vi "Initial_guess_gaussian_fit.vi"(10 "x-Axis in":dbl[](array[numeric]), 11 "Signal in":dbl[](array[numeric])) -> (0 "Initial guess FWHM":dbl, 1 "Initial guess Sigma":dbl, 2 "x-Axis out":dbl[](array[numeric]), 3 "Signal out":dbl[](array[numeric]), 4 "Parameter Bounds Cluster":T1, 5 "Initial Guess Cluster":T2, 6 "Initial guess Amplitude":dbl, 8 "Initial guess Offset":dbl)   [LabVIEW 2018]
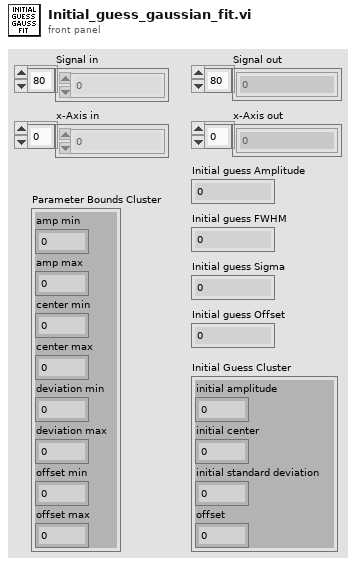
[diagram p1: front panel]
types:
  T1 = cluster{"amp min":dbl, "amp max":dbl, "center min":dbl, "center max":dbl, "deviation min":dbl, "deviation max":dbl, "offset min":dbl, "offset max":dbl}
  T2 = cluster{"initial amplitude":dbl, "initial center":dbl, "initial standard deviation":dbl, "offset":dbl}
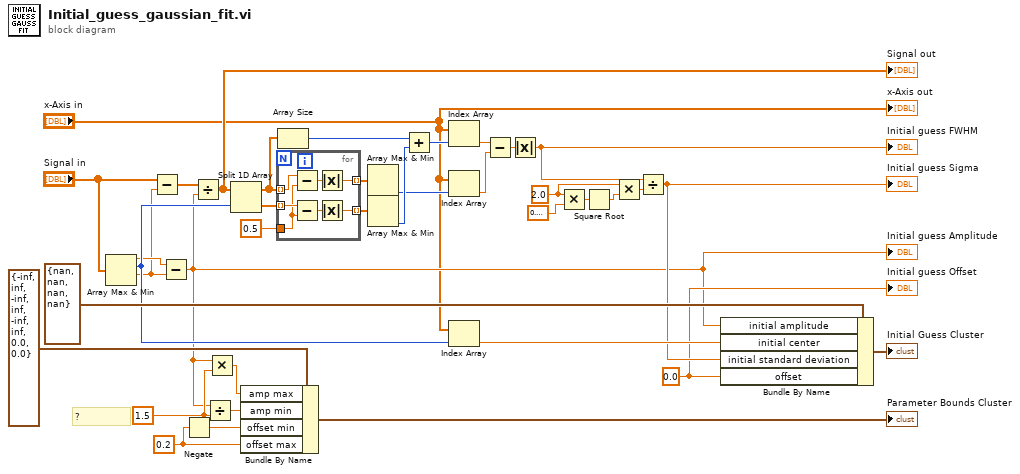
[diagram p0: block diagram]
diagram:
  w5 = 0.2 ("offset min")
  w8 = 1.5
  w11 = 0.0
  w36 = 2.0 ("x")
  # "?"
  n1 = Array Max & Min(array="Signal in") -> (max value=w14:dbl, max index (indices)=w20:i32, min value=w13:dbl)  [unwired: 1 out]
  n2 = Subtract(x="Signal in", y=w13) -> (x-y=w12:dbl[])
  n3 = Subtract(x=w14, y=w13) -> (x-y=w3:dbl)
  "Initial guess Amplitude" <- w3
  n4 = Negate(x=w5) -> (-x=w4:dbl)
  n5 = Divide(x=w12, y=w3) -> (x/y=w10:dbl[])
  "Signal out" <- w10
  n6 = Divide(x=w3, y=w8) -> (x/y=w7:dbl)
  n7 = Multiply(x=w3, y=w8) -> (x*y=w6:dbl)
  n8 = Split 1D Array(array=w10, index=w20) -> (first subarray=w24:dbl[], second subarray=w25:dbl[])
  n9 = Bundle By Name(cluster=T1 {"amp min"=-inf, "amp max"=inf, "center min"=-inf, "center max"=inf, "deviation min"=-inf, "deviation max"=inf, "offset min"=0.0, "offset max"=0.0} ("parameter bounds"), "amp max"=w6, "amp min"=w7, "offset min"=w4, "offset max"=w5) -> (→"Parameter Bounds Cluster":T1)
  n10 = for {
    tunnel: [w44] -> w33 mode=indexing
    tunnel: w24 -> [w42] mode=indexing
    tunnel: w25 -> [w41] mode=indexing
    tunnel: [w40] -> w32 mode=indexing
    tunnel: 0.5 -> [w39]
    n11 = Subtract(x=w42, y=w39) -> (x-y=w43:dbl)
    n12 = Subtract(x=w41, y=w39) -> (x-y=w45:dbl)
    n13 = Absolute Value(x=w43) -> (abs(x)=w40:dbl)
    n14 = Absolute Value(x=w45) -> (abs(x)=w44:dbl)
  }
  n15 = Array Size(array=w24) -> (size(s)=w29:i32)
  n16 = Array Max & Min(array=w32) -> (min index (indices)=w26:i32)  [unwired: 3 out]
  n17 = Array Max & Min(array=w33) -> (min index (indices)=w28:i32)  [unwired: 3 out]
  n18 = Add(x=w29, y=w28) -> (x+y=w27:i32)
  n19 = Index Array(array="x-Axis in", index=w27) -> (element=w22:dbl)
  n20 = Index Array(array="x-Axis in", index=w26) -> (element=w23:dbl)
  n21 = Index Array(array="x-Axis in", index=w20) -> (element=w19:dbl)
  n22 = Subtract(x=w22, y=w23) -> (x-y=w31:dbl)
  n23 = Absolute Value(x=w31) -> (abs(x)=w30:dbl)
  "Initial guess FWHM" <- w30
  n24 = Multiply(x=w36, y=0.6931471805599453) -> (x*y=w34:dbl)
  n25 = Square Root(x=w34) -> (sqrt(x)=w37:dbl)
  n26 = Multiply(x=w36, y=w37) -> (x*y=w38:dbl)
  n27 = Divide(x=w30, y=w38) -> (x/y=w18:dbl)
  "Initial guess Sigma" <- w18
  n28 = Bundle By Name(cluster=T2 {"initial amplitude"=nan, "initial center"=nan, "initial standard deviation"=nan, "offset"=nan} ("initial guess"), "initial amplitude"=w3, "initial center"=w19, "initial standard deviation"=w18, "offset"=w11) -> (→"Initial Guess Cluster":T2)
  "Initial guess Offset" <- w11
  "x-Axis out" <- "x-Axis in"
